vi "Wait for Operation Complete.vi"(8 "error in (no error)":errorcluster, 10 "Timeout (10000 ms)":u32=10000, 11 "VISA resource name":refnum<visa-resource-name>) -> (0 "error out":errorcluster, 3 "VISA resource name out":refnum<visa-resource-name>)   [LabVIEW 2009, in "Keithley 24XX.lvlib"]
doc: "Waits for an operation to complete. This is useful for synchronizing instrument code with other code.\n\n<B>Note:</B> When taking measurements, this VI will hold until the instrument has armed and triggered all of the times specified in Configure Multipoint. This VI won't function correctly if the triggering has occured but the instrument is set to arm after those triggered measurements have finished.\n\nUse this VI only with other low-level VIs. The high-level VIs automatically incorporate this functionality. This VI does not check the instrument status. If you want to check the instrument status, call the Error Query VI at the conclusion of the sequence."
uses:
  <instrlib>/Keithley 24XX/Keithley 24XX.lvlib
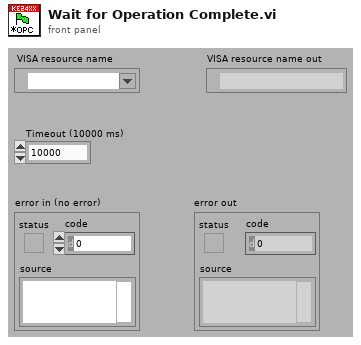
[diagram p1: front panel]
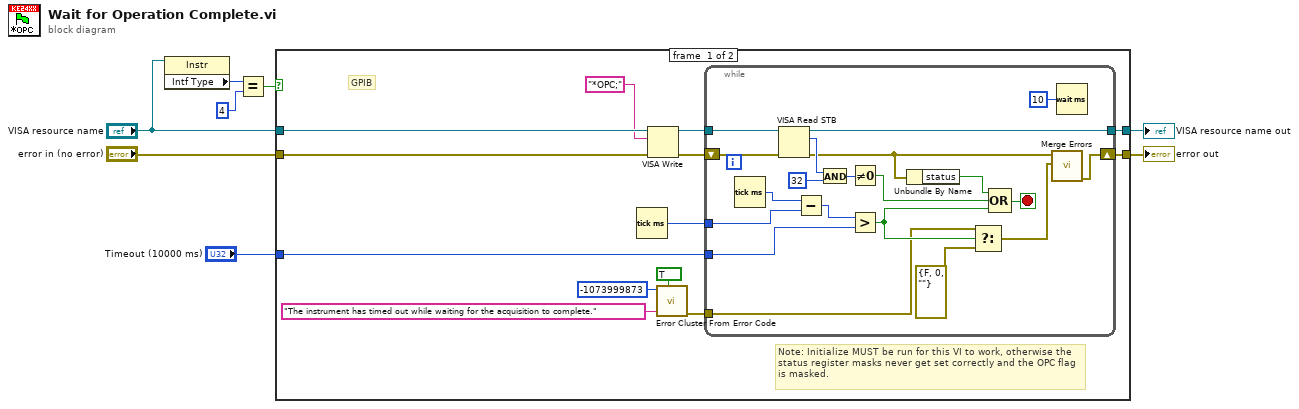
[diagram p0: block diagram]
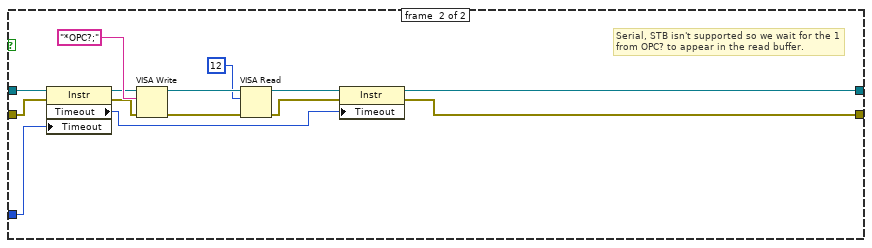
[diagram p2: hidden frame]
diagram:
  n1 = property class="Instr"(reference="VISA resource name") -> ("Intf Type"=w3:u16)  [unwired: 1 in, 2 out]
  n2 = Equal?(x=w3, y=u16 4) -> (x = y?=w4:bool)
  n3 = case shown="False" w4 {
    tunnel: "VISA resource name" -> [w21 w51]
    tunnel: "error in (no error)" -> [w20 w46]
    tunnel: [w17 w42] -> w7
    tunnel: [w16 w47] -> w6
    tunnel: "Timeout (10000 ms)" -> [w9 w50]
    frame #0 {
      # "GPIB"
      # "Note: Initialize MUST be run for this VI to work, otherwise the status register masks never get set correctly and the OPC flag is masked."
      n4 = Tick Count (ms)() -> (millisecond timer value=w14:u32)
      n5 = VISA Write(VISA resource name=w21, write buffer="*OPC;", error in (no error)=w20) -> (VISA resource name out=w19:refnum<visa-resource-name>, error out=w18:errorcluster)  [unwired: 1 out]
      n6 = call <vilib>:"Error Cluster From Error Code.vi"("show call chain? (False)"=TRUE, "error message (\"\")"="The instrument has timed out while waiting for the acquisition to complete." ("error message (\"\")"), "error code (0)"=-1073999873) -> ("error out"=w10:errorcluster)  [unwired: 6 in]
      n7 = while {
        tunnel: w19 -> [w41]
        tunnel: [w39] -> w16
        tunnel: w14 -> [w34]
        shift-right: [w26] -> w17
        shift-left: w18 -> [w40]
        tunnel: w10 -> [w29]
        tunnel: w9 -> [w22]
        stop <- w31 stop-if-true
        n8 = Tick Count (ms)() -> (millisecond timer value=w35:u32)
        n9 = VISA Read STB(8:w40, 11:w41) -> (0:w25:errorcluster, 2:w38:u16, 3:w39:refnum<visa-resource-name>)
        n10 = Subtract(x=w35, y=w34) -> (x-y=w33:u32)
        n11 = And(x=w38, y=u16 32) -> (x .and. y?=w36:u16)
        n12 = Not Equal To 0?(x=w36) -> (x != 0?=w32:bool)
        n13 = Greater?(x=w33, y=w22) -> (0:w30:bool)
        n14 = Unbundle By Name(w25) -> ("status"=w24:bool)
        n15 = Select(t=w29, s=w30, f=errorcluster {"status"=FALSE, "code"=0, "source"=""}) -> (s? t:f=w27:errorcluster)
        n16 = Compound Arithmetic op=OR(w24, w32, w30) -> (w31:bool)
        n17 = call <vilib>:"Merge Errors.vi"("error in 2 (no error)"=w27, "error in 1 (no error)"=w25) -> ("error out"=w26:errorcluster)  [unwired: 5 in]
        n18 = Wait (ms)(milliseconds to wait=u32 10) -> ()  [unwired: 1 out]
      }
    }
    frame #1 {
      # "Serial, STB isn't supported so we wait for the 1 \nfrom OPC? to appear in the read buffer."
      n19 = property class="Instr"(reference=w51, error in=w46, "Timeout"=w50) -> (reference out=w45:refnum<visa-resource-name>, error out=w44:errorcluster, "Timeout"=w49:u32)
      n20 = VISA Write(VISA resource name=w45, write buffer="*OPC?;", error in (no error)=w44) -> (VISA resource name out=w53:refnum<visa-resource-name>, error out=w54:errorcluster)  [unwired: 1 out]
      n21 = VISA Read(VISA resource name=w53, byte count=u32 12, error in (no error)=w54) -> (VISA resource name out=w48:refnum<visa-resource-name>, error out=w43:errorcluster)  [unwired: 2 out]
      n22 = property class="Instr"(reference=w48, error in=w43, "Timeout"=w49) -> (reference out=w47:refnum<visa-resource-name>, error out=w42:errorcluster)
    }
  }
  "VISA resource name out" <- w6
  "error out" <- w7
